vi "Ballard XML Generator.Add Raw Data.vi"(10 "raw data":string, 11 "string in":string) -> (3 "string out":string)   [LabVIEW 2020]
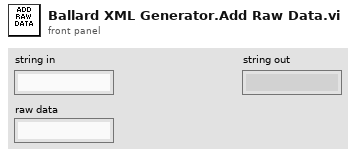
[diagram p1: front panel]
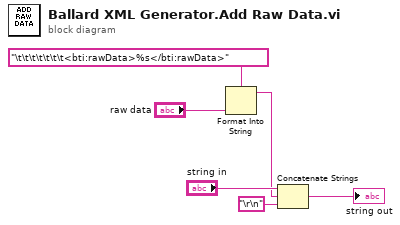
[diagram p0: block diagram]
diagram:
  n1 = Format Into String(format string="\t\t\t\t\t\t\t<bti:rawData>%s</bti:rawData>", "raw data") -> (resulting string=w2:string)  [unwired: 2 in, 1 out]
  n2 = Concatenate Strings("string in", w2, "\r\n") -> (→"string out":string)
